vi "RT Loop - UI Commands.vi"(11 "Message Queue":refnum<queue>) -> ()   [LabVIEW 2020]
doc: "Use this template to build a simple state machine design pattern. Each state executes code and determines which state to transition to."
uses:
  support/Message Queue/Message Cluster.ctl
  controls/RT Loop - UI Communication State.ctl
  Globals/Global - Configuration Options.vi
  Globals/Global - All RT Loop Stop.vi
  Globals/Global - RT Stream Connections.vi
  support/Message Queue/Message Queue.lvlib
  <resource>/objmgr/ni.dex.rc
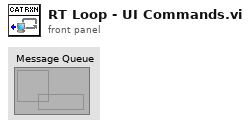
[diagram p1: front panel]
types:
  T1 = typedef "RT Loop - UI Communication State.ctl" = enum16{"Initialize", "Listen for UI Writer", "Receive UI Commands"}
  T2 = typedef "Message Queue.lvlib/Message Cluster.ctl" = cluster{"Message":string, "Message Data":variant}
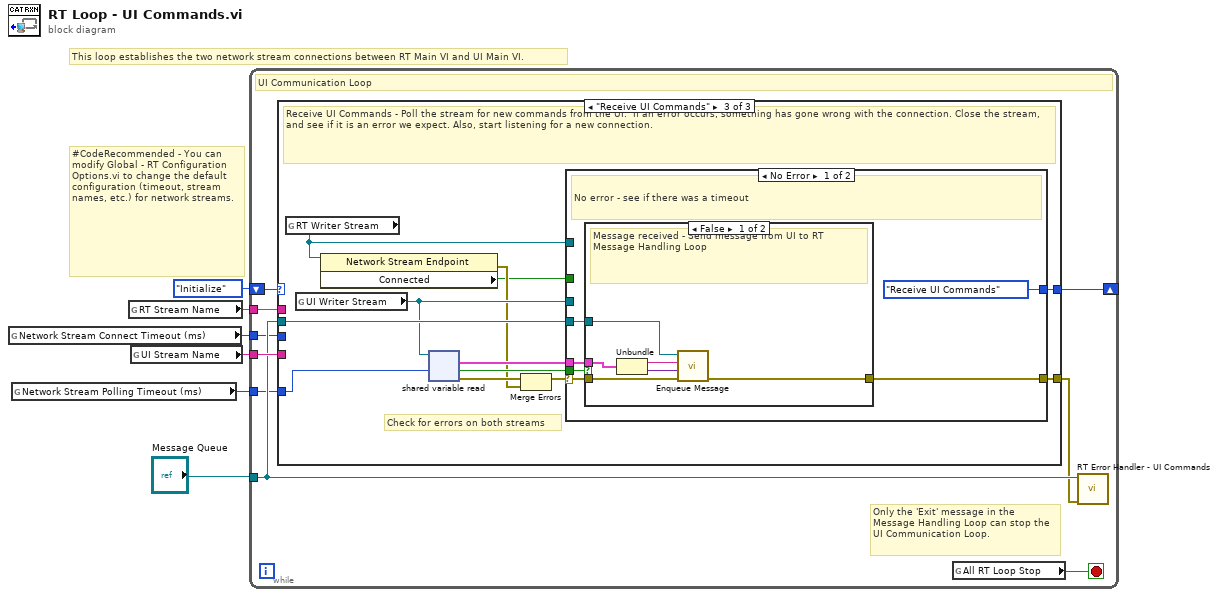
[diagram p0: block diagram]
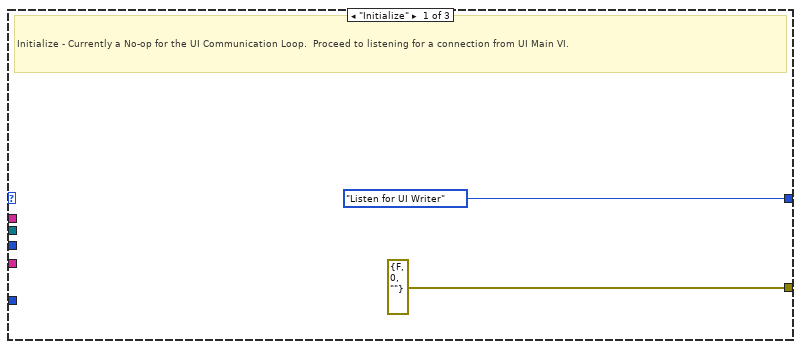
[diagram p2: hidden frame]
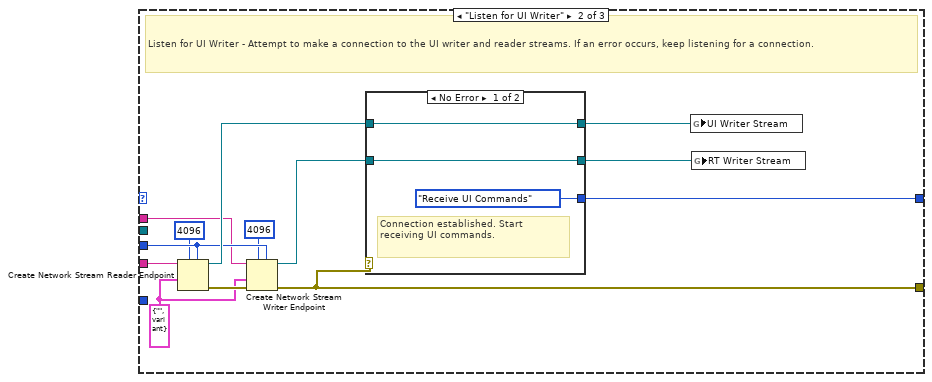
[diagram p3: hidden frame]
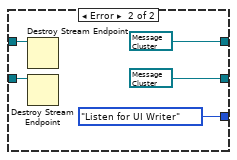
[diagram p4: hidden frame]
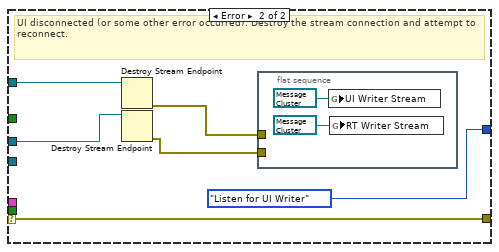
[diagram p6: hidden frame]
diagram:
  # "#CodeRecommended - You can modify Global - RT Configuration Options.vi to change the default configuration (timeout, stream names, etc.) for network streams."
  # "This loop establishes the two network stream connections between RT Main VI and UI Main VI."
  n1 = global read "Global - Configuration Options.vi" "Network Stream Connect Timeout (ms)"() -> (w1:i32)
  n2 = global read "Global - Configuration Options.vi" "Network Stream Polling Timeout (ms)"() -> (w2:i32)
  n3 = global read "Global - Configuration Options.vi" "RT Stream Name"() -> (w3:string)
  n4 = global read "Global - Configuration Options.vi" "UI Stream Name"() -> (w4:string)
  n5 = while {
    shift-right: [w14] -> _
    shift-left: RT_Loop_-_UI_Communication_State."Initialize" ("RT Loop - Host Communication State") -> [w15]
    tunnel: "Message Queue" -> [w11]
    tunnel: w4 -> [w12]
    tunnel: w3 -> [w9]
    tunnel: w2 -> [w8]
    tunnel: w1 -> [w7]
    stop <- w13 stop-if-true
    # "Only the 'Exit' message in the  Message Handling Loop can stop the UI Communication Loop."
    # "UI Communication Loop"
    n6 = case shown="\"Receive UI Commands\"" w15 {
      tunnel: [RT_Loop_-_UI_Communication_State."Listen for UI Writer" ("RT Loop - Host Communication State") w29 w49] -> w14
      tunnel: [errorcluster {"status"=FALSE, "code"=0, "source"=""} ("error IO") w24 w50] -> w10
      tunnel: w7 -> [_ w23 _]
      tunnel: w12 -> [_ w28 _]
      tunnel: w11 -> [_ _ w48]
      tunnel: w9 -> [_ w22 _]
      tunnel: w8 -> [_ _ w39]
      frame "Initialize" {
        # "Initialize - Currently a No-op for the UI Communication Loop.  Proceed to listening for a connection from UI Main VI."
      }
      frame "Listen for UI Writer" {
        w26 = T2 {"Message"="", "Message Data"=variant} ("Message Cluster")
        # "Listen for UI Writer - Attempt to make a connection to the UI writer and reader streams. If an error occurs, keep listening for a connection."
        n7 = Create Network Stream Reader Endpoint(5:w23, 7:4096 ("reader buffer size"), 9:w26, 11:w28) -> (0:w27:errorcluster, 3:w30:refnum<k21>)  [unwired: 3 in]
        n8 = Create Network Stream Writer Endpoint(5:w23, 7:4096 ("writer buffer size"), 8:w27, 9:w26, 11:w22) -> (0:w24:errorcluster, 3:w25:refnum<k21>)  [unwired: 2 in]
        n9 = case shown="No Error" w24 {
          tunnel: w30 -> [w32 w35]
          tunnel: [RT_Loop_-_UI_Communication_State."Receive UI Commands" ("RT Loop - Host Communication State") RT_Loop_-_UI_Communication_State."Listen for UI Writer" ("RT Loop - Host Communication State")] -> w29
          tunnel: w25 -> [w31 w34]
          tunnel: [w32 refnum<k21> refnum] -> w21
          tunnel: [w31 refnum<k21> refnum] -> w20
          frame No Error {
            # "Connection established. Start receiving UI commands."
          }
          frame Error {
            n10 = Destroy Stream Endpoint(11:w35) -> ()  [unwired: 1 in, 1 out]
            n11 = Destroy Stream Endpoint(11:w34) -> ()  [unwired: 1 in, 1 out]
          }
        }
        n12 = global write "Global - RT Stream Connections.vi" "UI Writer Stream"(w21) -> ()
        n13 = global write "Global - RT Stream Connections.vi" "RT Writer Stream"(w20) -> ()
      }
      frame "Receive UI Commands" {
        # "Check for errors on both streams"
        # "Receive UI Commands - Poll the stream for new commands from the UI.  If an error occurs, something has gone wrong with the connection. Close the stream, and see if it is an error we expect. Also, start listening for a new connection."
        n14 = global read "Global - RT Stream Connections.vi" "RT Writer Stream"() -> (w40:refnum<k21>)
        n15 = global read "Global - RT Stream Connections.vi" "UI Writer Stream"() -> (w44:refnum<k21>)
        n16 = property class="Network Stream Endpoint"(reference=w40) -> (error out=w42:errorcluster, "Connected"=w41:bool)  [unwired: 1 in, 1 out]
        n17 = shared-variable-read(w44, w39) -> (w45:errorcluster, w46:bool, w47:T2)  [unwired: 1 in, 1 out]
        n18 = Merge Errors(w45, w42) -> (w43:errorcluster)
        n19 = case shown="No Error" w43 {
          selector: w43 -> [w54 w68]
          tunnel: [w53 w68] -> w50
          tunnel: w46 -> [w56 _]
          tunnel: w47 -> [w55 _]
          tunnel: [RT_Loop_-_UI_Communication_State."Receive UI Commands" ("RT Loop - Host Communication State") RT_Loop_-_UI_Communication_State."Listen for UI Writer" ("RT Loop - Host Communication State")] -> w49
          tunnel: w48 -> [w52 _]
          tunnel: w44 -> [_ w65]
          tunnel: w41 -> [_ _]
          tunnel: w40 -> [_ w64]
          frame No Error {
            # "No error - see if there was a timeout"
            n20 = case shown="False" w56 {
              tunnel: w55 -> [w61 _]
              tunnel: w54 -> [w62 w63]
              tunnel: [w57 w63] -> w53
              tunnel: w52 -> [w58 _]
              frame False {
                # "Message received - Send message from UI to RT Message Handling Loop"
                n21 = Unbundle(w61) -> ("Message"=w60:string, "Message Data"=w59:variant)
                n22 = call "Enqueue Message.vi"("error in (no error)"=w62, "Message Data"=w59, "Message"=w60, "Message Queue"=w58) -> ("error out"=w57:errorcluster)  [unwired: 6 in, 1 out]
              }
              frame True {
                # "Timeout - no new command"
              }
            }
          }
          frame Error {
            # "UI disconnected (or some other error occurred). Destroy the stream connection and attempt to reconnect."
            n23 = Destroy Stream Endpoint(11:w64) -> (0:w67:errorcluster)  [unwired: 1 in]
            n24 = Destroy Stream Endpoint(11:w65) -> (0:w66:errorcluster)  [unwired: 1 in]
            n25 = flat-sequence {
              tunnel: w67 -> [_]
              tunnel: w66 -> [_]
              frame #0 {
                n26 = global write "Global - RT Stream Connections.vi" "UI Writer Stream"(refnum<k21> refnum ("Host Writer Stream")) -> ()
                n27 = global write "Global - RT Stream Connections.vi" "RT Writer Stream"(refnum<k21> refnum ("RT Writer Stream")) -> ()
              }
            }
          }
        }
      }
    }
    n28 = global read "Global - All RT Loop Stop.vi" "All RT Loop Stop"() -> (w13:bool)
    n29 = call "RT Error Handler - UI Commands.vi"("error in (no error)"=w10, "Message Queue"=w11) -> ()  [unwired: 9 in, 1 out]
  }
